vi "SPAN Stufen Gasteiler testen.vi"(5 "Stufen Tabelle Array":string[][][](array[string]), 6 "Sprachliste":string[][](array[string]), 7 "Boolsche Stufen Flags Cluster":T11, 8 "error in (no error)":errorcluster caption="Fehler (Eingang, kein Fehler)", 9 "Index":T13, 10 "Referenzen Cluster":T12, 11 "SpanInletClusterArray in":T2[](array[typedef]) {"zusätzliche Zeitdauer Erster Punkt" min=30 step=1 format="%#_5g"; "Zeitdauer Stufen" format="%#_5g"; "Max Fehler" format="%#_5g"; "Anzahl Stufen" format="%#_5g"; "Komponenten"."Komponente 5"."Komponente:" items=["NO (350,3000) LP 191C", "NO2 (150) LP 191C (1of2)", "NO2 (2000) LP 191C (2of2)", "N2O (300) LP 191C (1of2)", "NH3 (300) LP 191C (1of2)", "NH3 (900,3000) LP 191C (2of2)", "HNCO (400) 191C", "H2O% (30) LP 191C", "Formaldehyde (70,500) LP 191C", "CO2 low% (4) LP 191C (2of2)", "CO2% (20) LP 191C (1of2)", "CO (700) LP 191C (1of3)", "CO% (1) LP 191C (2of3)", "Propylene (1000) LP 191C", "Aromatic HC C7 (500) LP 191C", "Ethylene (1000) LP 191C", "CH4 (250) LP 191C (1of2)", "CH4 (5000) LP 191C (2of2)", "Ethane (1000) LP 191C", "Acetylene (1000) LP 191C", "HNO2 (20) 191C", "MeOH (1000) 191C", "CO% (10) LP 191C (3of3)", "Formic Acid (100) 191C", "SO2 (500) LP 191C", "Acetaldehyde (1000) LP 191C", "COS (100) LP 191C", "1,3 butadiene (100) LP 191C", "Oil as Octane (200) LP 191C", "N2O (1000) LP 191C (2of2)", "Propane (200) LP 191C", "NO2 autorange (2000)", "CO autorange (100000)", "CH4 autorange (5000)", "NH3 autorange (3000)", "Temp. Gascell", "Pressure Gascell", "sBeam@2500"]; "Komponenten"."Komponente 5"."Konzentration IST" format="%#.4f"; "Komponenten"."Komponente 5"."Genauigkeit" format="%#.1f"; "Komponenten"."Komponente 4"."Komponente:" items=["NO (350,3000) LP 191C", "NO2 (150) LP 191C (1of2)", "NO2 (2000) LP 191C (2of2)", "N2O (300) LP 191C (1of2)", "NH3 (300) LP 191C (1of2)", "NH3 (900,3000) LP 191C (2of2)", "HNCO (400) 191C", "H2O% (30) LP 191C", "Formaldehyde (70,500) LP 191C", "CO2 low% (4) LP 191C (2of2)", "CO2% (20) LP 191C (1of2)", "CO (700) LP 191C (1of3)", "CO% (1) LP 191C (2of3)", "Propylene (1000) LP 191C", "Aromatic HC C7 (500) LP 191C", "Ethylene (1000) LP 191C", "CH4 (250) LP 191C (1of2)", "CH4 (5000) LP 191C (2of2)", "Ethane (1000) LP 191C", "Acetylene (1000) LP 191C", "HNO2 (20) 191C", "MeOH (1000) 191C", "CO% (10) LP 191C (3of3)", "Formic Acid (100) 191C", "SO2 (500) LP 191C", "Acetaldehyde (1000) LP 191C", "COS (100) LP 191C", "1,3 butadiene (100) LP 191C", "Oil as Octane (200) LP 191C", "N2O (1000) LP 191C (2of2)", "Propane (200) LP 191C", "NO2 autorange (2000)", "CO autorange (100000)", "CH4 autorange (5000)", "NH3 autorange (3000)", "Temp. Gascell", "Pressure Gascell", "sBeam@2500"]; "Komponenten"."Komponente 4"."Konzentration IST" format="%#.4f"; "Komponenten"."Komponente 4"."Genauigkeit" format="%#.1f"; "Komponenten"."Komponente 3"."Komponente:" items=["NO (350,3000) LP 191C", "NO2 (150) LP 191C (1of2)", "NO2 (2000) LP 191C (2of2)", "N2O (300) LP 191C (1of2)", "NH3 (300) LP 191C (1of2)", "NH3 (900,3000) LP 191C (2of2)", "HNCO (400) 191C", "H2O% (30) LP 191C", "Formaldehyde (70,500) LP 191C", "CO2 low% (4) LP 191C (2of2)", "CO2% (20) LP 191C (1of2)", "CO (700) LP 191C (1of3)", "CO% (1) LP 191C (2of3)", "Propylene (1000) LP 191C", "Aromatic HC C7 (500) LP 191C", "Ethylene (1000) LP 191C", "CH4 (250) LP 191C (1of2)", "CH4 (5000) LP 191C (2of2)", "Ethane (1000) LP 191C", "Acetylene (1000) LP 191C", "HNO2 (20) 191C", "MeOH (1000) 191C", "CO% (10) LP 191C (3of3)", "Formic Acid (100) 191C", "SO2 (500) LP 191C", "Acetaldehyde (1000) LP 191C", "COS (100) LP 191C", "1,3 butadiene (100) LP 191C", "Oil as Octane (200) LP 191C", "N2O (1000) LP 191C (2of2)", "Propane (200) LP 191C", "NO2 autorange (2000)", "CO autorange (100000)", "CH4 autorange (5000)", "NH3 autorange (3000)", "Temp. Gascell", "Pressure Gascell", "sBeam@2500"]; "Komponenten"."Komponente 3"."Konzentration IST" format="%#.4f"; "Komponenten"."Komponente 3"."Genauigkeit" format="%#.1f"; "Komponenten"."Komponente 2"."Komponente:" items=["NO (350,3000) LP 191C", "NO2 (150) LP 191C (1of2)", "NO2 (2000) LP 191C (2of2)", "N2O (300) LP 191C (1of2)", "NH3 (300) LP 191C (1of2)", "NH3 (900,3000) LP 191C (2of2)", "HNCO (400) 191C", "H2O% (30) LP 191C", "Formaldehyde (70,500) LP 191C", "CO2 low% (4) LP 191C (2of2)", "CO2% (20) LP 191C (1of2)", "CO (700) LP 191C (1of3)", "CO% (1) LP 191C (2of3)", "Propylene (1000) LP 191C", "Aromatic HC C7 (500) LP 191C", "Ethylene (1000) LP 191C", "CH4 (250) LP 191C (1of2)", "CH4 (5000) LP 191C (2of2)", "Ethane (1000) LP 191C", "Acetylene (1000) LP 191C", "HNO2 (20) 191C", "MeOH (1000) 191C", "CO% (10) LP 191C (3of3)", "Formic Acid (100) 191C", "SO2 (500) LP 191C", "Acetaldehyde (1000) LP 191C", "COS (100) LP 191C", "1,3 butadiene (100) LP 191C", "Oil as Octane (200) LP 191C", "N2O (1000) LP 191C (2of2)", "Propane (200) LP 191C", "NO2 autorange (2000)", "CO autorange (100000)", "CH4 autorange (5000)", "NH3 autorange (3000)", "Temp. Gascell", "Pressure Gascell", "sBeam@2500"]; "Komponenten"."Komponente 2"."Konzentration IST" format="%#.4f"; "Komponenten"."Komponente 2"."Genauigkeit" format="%#.1f"; "Komponenten"."Komponente 1"."Komponente:" items=["NO (350,3000) LP 191C", "NO2 (150) LP 191C (1of2)", "NO2 (2000) LP 191C (2of2)", "N2O (300) LP 191C (1of2)", "NH3 (300) LP 191C (1of2)", "NH3 (900,3000) LP 191C (2of2)", "HNCO (400) 191C", "H2O% (30) LP 191C", "Formaldehyde (70,500) LP 191C", "CO2 low% (4) LP 191C (2of2)", "CO2% (20) LP 191C (1of2)", "CO (700) LP 191C (1of3)", "CO% (1) LP 191C (2of3)", "Propylene (1000) LP 191C", "Aromatic HC C7 (500) LP 191C", "Ethylene (1000) LP 191C", "CH4 (250) LP 191C (1of2)", "CH4 (5000) LP 191C (2of2)", "Ethane (1000) LP 191C", "Acetylene (1000) LP 191C", "HNO2 (20) 191C", "MeOH (1000) 191C", "CO% (10) LP 191C (3of3)", "Formic Acid (100) 191C", "SO2 (500) LP 191C", "Acetaldehyde (1000) LP 191C", "COS (100) LP 191C", "1,3 butadiene (100) LP 191C", "Oil as Octane (200) LP 191C", "N2O (1000) LP 191C (2of2)", "Propane (200) LP 191C", "NO2 autorange (2000)", "CO autorange (100000)", "CH4 autorange (5000)", "NH3 autorange (3000)", "Temp. Gascell", "Pressure Gascell", "sBeam@2500"]; "Komponenten"."Komponente 1"."Konzentration IST" format="%#.4f"; "Komponenten"."Komponente 1"."Genauigkeit" format="%#.1f"; "Ablaufdatum" format="%<%d.%m.%Y>T"; "Gasflasche" items=["----"=10000, "IAG NH3 3000"=0, "IAG NH3 200"=1, "IAG NH3 2000"=2, "IAG MG"=3, "IAG O2"=4]}) -> (0 "error out":errorcluster caption="Fehler (Ausgang)", 1 "GD LNI old or other":T1 caption="GD LNI old", 2 "GD DF":T1, 3 "SpanInletClusterArray out":T2[](array[typedef]) {"zusätzliche Zeitdauer Erster Punkt" min=30 step=1 format="%#_5g"; "Zeitdauer Stufen" format="%#_5g"; "Max Fehler" format="%#_5g"; "Anzahl Stufen" format="%#_5g"; "Komponenten"."Komponente 5"."Komponente:" items=["NO (350,3000) LP 191C", "NO2 (150) LP 191C (1of2)", "NO2 (2000) LP 191C (2of2)", "N2O (300) LP 191C (1of2)", "NH3 (300) LP 191C (1of2)", "NH3 (900,3000) LP 191C (2of2)", "HNCO (400) 191C", "H2O% (30) LP 191C", "Formaldehyde (70,500) LP 191C", "CO2 low% (4) LP 191C (2of2)", "CO2% (20) LP 191C (1of2)", "CO (700) LP 191C (1of3)", "CO% (1) LP 191C (2of3)", "Propylene (1000) LP 191C", "Aromatic HC C7 (500) LP 191C", "Ethylene (1000) LP 191C", "CH4 (250) LP 191C (1of2)", "CH4 (5000) LP 191C (2of2)", "Ethane (1000) LP 191C", "Acetylene (1000) LP 191C", "HNO2 (20) 191C", "MeOH (1000) 191C", "CO% (10) LP 191C (3of3)", "Formic Acid (100) 191C", "SO2 (500) LP 191C", "Acetaldehyde (1000) LP 191C", "COS (100) LP 191C", "1,3 butadiene (100) LP 191C", "Oil as Octane (200) LP 191C", "N2O (1000) LP 191C (2of2)", "Propane (200) LP 191C", "NO2 autorange (2000)", "CO autorange (100000)", "CH4 autorange (5000)", "NH3 autorange (3000)", "Temp. Gascell", "Pressure Gascell", "sBeam@2500"]; "Komponenten"."Komponente 5"."Konzentration IST" format="%#.4f"; "Komponenten"."Komponente 5"."Genauigkeit" format="%#.1f"; "Komponenten"."Komponente 4"."Komponente:" items=["NO (350,3000) LP 191C", "NO2 (150) LP 191C (1of2)", "NO2 (2000) LP 191C (2of2)", "N2O (300) LP 191C (1of2)", "NH3 (300) LP 191C (1of2)", "NH3 (900,3000) LP 191C (2of2)", "HNCO (400) 191C", "H2O% (30) LP 191C", "Formaldehyde (70,500) LP 191C", "CO2 low% (4) LP 191C (2of2)", "CO2% (20) LP 191C (1of2)", "CO (700) LP 191C (1of3)", "CO% (1) LP 191C (2of3)", "Propylene (1000) LP 191C", "Aromatic HC C7 (500) LP 191C", "Ethylene (1000) LP 191C", "CH4 (250) LP 191C (1of2)", "CH4 (5000) LP 191C (2of2)", "Ethane (1000) LP 191C", "Acetylene (1000) LP 191C", "HNO2 (20) 191C", "MeOH (1000) 191C", "CO% (10) LP 191C (3of3)", "Formic Acid (100) 191C", "SO2 (500) LP 191C", "Acetaldehyde (1000) LP 191C", "COS (100) LP 191C", "1,3 butadiene (100) LP 191C", "Oil as Octane (200) LP 191C", "N2O (1000) LP 191C (2of2)", "Propane (200) LP 191C", "NO2 autorange (2000)", "CO autorange (100000)", "CH4 autorange (5000)", "NH3 autorange (3000)", "Temp. Gascell", "Pressure Gascell", "sBeam@2500"]; "Komponenten"."Komponente 4"."Konzentration IST" format="%#.4f"; "Komponenten"."Komponente 4"."Genauigkeit" format="%#.1f"; "Komponenten"."Komponente 3"."Komponente:" items=["NO (350,3000) LP 191C", "NO2 (150) LP 191C (1of2)", "NO2 (2000) LP 191C (2of2)", "N2O (300) LP 191C (1of2)", "NH3 (300) LP 191C (1of2)", "NH3 (900,3000) LP 191C (2of2)", "HNCO (400) 191C", "H2O% (30) LP 191C", "Formaldehyde (70,500) LP 191C", "CO2 low% (4) LP 191C (2of2)", "CO2% (20) LP 191C (1of2)", "CO (700) LP 191C (1of3)", "CO% (1) LP 191C (2of3)", "Propylene (1000) LP 191C", "Aromatic HC C7 (500) LP 191C", "Ethylene (1000) LP 191C", "CH4 (250) LP 191C (1of2)", "CH4 (5000) LP 191C (2of2)", "Ethane (1000) LP 191C", "Acetylene (1000) LP 191C", "HNO2 (20) 191C", "MeOH (1000) 191C", "CO% (10) LP 191C (3of3)", "Formic Acid (100) 191C", "SO2 (500) LP 191C", "Acetaldehyde (1000) LP 191C", "COS (100) LP 191C", "1,3 butadiene (100) LP 191C", "Oil as Octane (200) LP 191C", "N2O (1000) LP 191C (2of2)", "Propane (200) LP 191C", "NO2 autorange (2000)", "CO autorange (100000)", "CH4 autorange (5000)", "NH3 autorange (3000)", "Temp. Gascell", "Pressure Gascell", "sBeam@2500"]; "Komponenten"."Komponente 3"."Konzentration IST" format="%#.4f"; "Komponenten"."Komponente 3"."Genauigkeit" format="%#.1f"; "Komponenten"."Komponente 2"."Komponente:" items=["NO (350,3000) LP 191C", "NO2 (150) LP 191C (1of2)", "NO2 (2000) LP 191C (2of2)", "N2O (300) LP 191C (1of2)", "NH3 (300) LP 191C (1of2)", "NH3 (900,3000) LP 191C (2of2)", "HNCO (400) 191C", "H2O% (30) LP 191C", "Formaldehyde (70,500) LP 191C", "CO2 low% (4) LP 191C (2of2)", "CO2% (20) LP 191C (1of2)", "CO (700) LP 191C (1of3)", "CO% (1) LP 191C (2of3)", "Propylene (1000) LP 191C", "Aromatic HC C7 (500) LP 191C", "Ethylene (1000) LP 191C", "CH4 (250) LP 191C (1of2)", "CH4 (5000) LP 191C (2of2)", "Ethane (1000) LP 191C", "Acetylene (1000) LP 191C", "HNO2 (20) 191C", "MeOH (1000) 191C", "CO% (10) LP 191C (3of3)", "Formic Acid (100) 191C", "SO2 (500) LP 191C", "Acetaldehyde (1000) LP 191C", "COS (100) LP 191C", "1,3 butadiene (100) LP 191C", "Oil as Octane (200) LP 191C", "N2O (1000) LP 191C (2of2)", "Propane (200) LP 191C", "NO2 autorange (2000)", "CO autorange (100000)", "CH4 autorange (5000)", "NH3 autorange (3000)", "Temp. Gascell", "Pressure Gascell", "sBeam@2500"]; "Komponenten"."Komponente 2"."Konzentration IST" format="%#.4f"; "Komponenten"."Komponente 2"."Genauigkeit" format="%#.1f"; "Komponenten"."Komponente 1"."Komponente:" items=["NO (350,3000) LP 191C", "NO2 (150) LP 191C (1of2)", "NO2 (2000) LP 191C (2of2)", "N2O (300) LP 191C (1of2)", "NH3 (300) LP 191C (1of2)", "NH3 (900,3000) LP 191C (2of2)", "HNCO (400) 191C", "H2O% (30) LP 191C", "Formaldehyde (70,500) LP 191C", "CO2 low% (4) LP 191C (2of2)", "CO2% (20) LP 191C (1of2)", "CO (700) LP 191C (1of3)", "CO% (1) LP 191C (2of3)", "Propylene (1000) LP 191C", "Aromatic HC C7 (500) LP 191C", "Ethylene (1000) LP 191C", "CH4 (250) LP 191C (1of2)", "CH4 (5000) LP 191C (2of2)", "Ethane (1000) LP 191C", "Acetylene (1000) LP 191C", "HNO2 (20) 191C", "MeOH (1000) 191C", "CO% (10) LP 191C (3of3)", "Formic Acid (100) 191C", "SO2 (500) LP 191C", "Acetaldehyde (1000) LP 191C", "COS (100) LP 191C", "1,3 butadiene (100) LP 191C", "Oil as Octane (200) LP 191C", "N2O (1000) LP 191C (2of2)", "Propane (200) LP 191C", "NO2 autorange (2000)", "CO autorange (100000)", "CH4 autorange (5000)", "NH3 autorange (3000)", "Temp. Gascell", "Pressure Gascell", "sBeam@2500"]; "Komponenten"."Komponente 1"."Konzentration IST" format="%#.4f"; "Komponenten"."Komponente 1"."Genauigkeit" format="%#.1f"; "Ablaufdatum" format="%<%d.%m.%Y>T"; "Gasflasche" items=["----"=10000, "IAG NH3 3000"=0, "IAG NH3 200"=1, "IAG NH3 2000"=2, "IAG MG"=3, "IAG O2"=4]})   [LabVIEW 2020, in "Linearisierung v2.lvlib" / "SpanEinstellungen.lvlib"]
uses:
  SpanEinstellungen.lvlib
  GD Abfrage Referenzen.ctl
  Boolsche Stufen Flags.ctl
  SpanInletCluster.ctl
  Seiten/System Einstellungen V2/Konfig Gasflasche.ctl
  Seiten/System Einstellungen V2/Analysatoren.ctl
  Seiten/System Einstellungen V2/Gasflasche Auswahl.ctl
  Komponentencluster mit Formel.ctl
  Komponentenauswahl mit Formel.ctl
  Visualisierungs Elemente/String - Eingabefeld.ctl
  Einheit.ctl
  Seiten/System Einstellungen V2/Traegergas.ctl
  Visualisierungs Elemente/Checkbox(boolsch).ctl
  Gasteiler/Aktionen FGV Gasteiler Daten.ctl
  GasteilerType.ctl
  Linearisierung v2.lvlib
  Gasteiler/Gasteiler.lvlib
  Sprachverwaltung/Sprachverwaltung.lvlib
  Seiten/System Einstellungen V2/System Einstellungen V2.lvlib
panel:
  # "sec"
  # "%"
  # "sec"
  # "Komponente"
  # "Formel"
  # "Konzentration"
  # "Einheit"
  # "Genauigkeit [%]"
  # "sec"
  # "%"
  # "sec"
  # "Komponente"
  # "Formel"
  # "Konzentration"
  # "Einheit"
  # "Genauigkeit [%]"
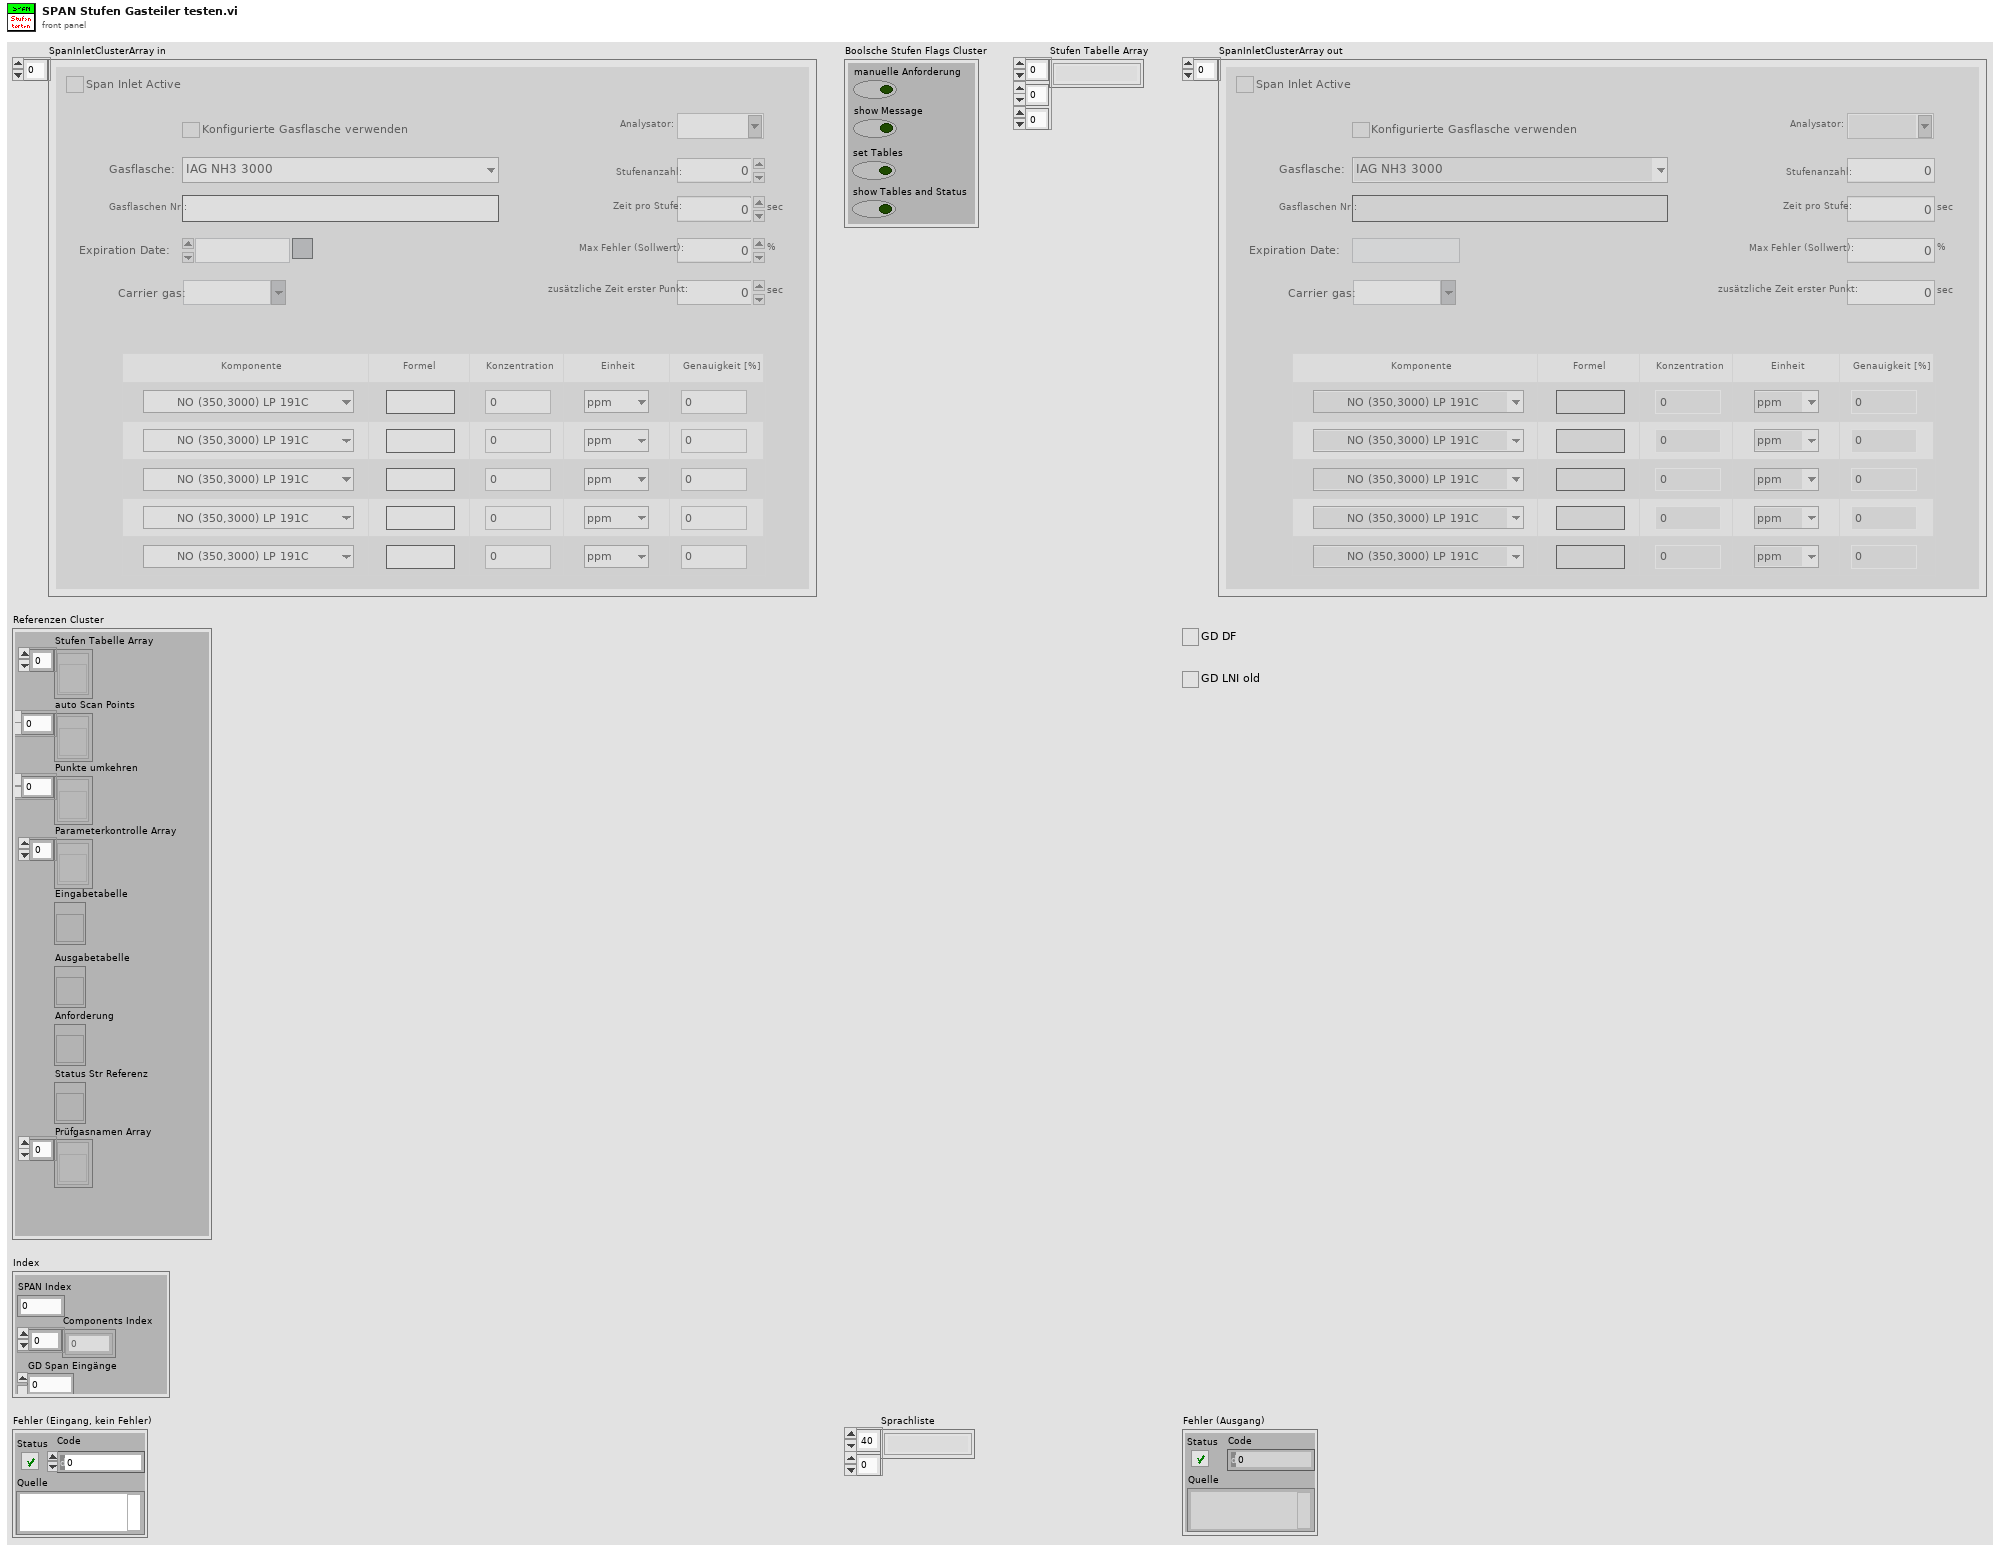
[diagram p1: front panel]
types:
  T1 = typedef "Checkbox(boolsch).ctl" = bool
  T2 = typedef "Linearisierung v2.lvlib/SpanEinstellungen.lvlib/SpanInletCluster.ctl" = cluster{"Span Inlet Active":T3, "Analysator":T4, "Konfig Gasflasche":T3, "Gasflasche":T5, "Gasflaschen Nr.:":string, "Ablaufdatum":timestamp, "Komponenten":T6, "Zeitdauer Stufen":sgl, "Max Fehler":sgl, "Anzahl Stufen":sgl, "Trägergas":T10, "zusätzliche Zeitdauer Erster Punkt":sgl}
  T3 = typedef "System Einstellungen V2.lvlib/Konfig Gasflasche.ctl" = bool
  T4 = typedef "System Einstellungen V2.lvlib/Analysatoren.ctl" = string
  T5 = typedef "System Einstellungen V2.lvlib/Gasflasche Auswahl.ctl" = u16
  T6 = typedef "Linearisierung v2.lvlib/SpanEinstellungen.lvlib/Komponentencluster mit Formel.ctl" = cluster{"Komponente 1":T7, "Komponente 2":T7, "Komponente 3":T7, "Komponente 4":T7, "Komponente 5":T7}
  T7 = typedef "Linearisierung v2.lvlib/SpanEinstellungen.lvlib/Komponentenauswahl mit Formel.ctl" = cluster{"Komponente:":u16, "Summenformel":T8, "Konzentration IST":dbl, "Einheit":T9, "Genauigkeit":dbl}
  T8 = typedef "String - Eingabefeld.ctl" = string
  T9 = typedef "Linearisierung v2.lvlib/SpanEinstellungen.lvlib/Einheit.ctl" = enum16{"ppm", "%"}
  T10 = typedef "System Einstellungen V2.lvlib/Traegergas.ctl" = string
  T11 = typedef "Linearisierung v2.lvlib/SpanEinstellungen.lvlib/Boolsche Stufen Flags.ctl" = cluster{"manuelle Anforderung":bool, "show Message":bool, "set Tables":bool, "show Tables and Status":bool}
  T12 = typedef "Linearisierung v2.lvlib/SpanEinstellungen.lvlib/GD Abfrage Referenzen.ctl" = cluster{"Stufen Tabelle Array":refnum<vi>[], "auto Scan Points":refnum<vi>[], "Punkte umkehren":refnum<vi>[], "Parameterkontrolle Array":refnum<vi>[], "Eingabetabelle":refnum<vi>, "Ausgabetabelle":refnum<vi>, "Anforderung":refnum<vi>, "Status Str Referenz":refnum<vi>, "Prüfgasnamen Array":refnum<vi>[]}
  T13 = cluster{"SPAN Index":i32, "Components Index":i32[], "GD Span Eingänge":u16}
  T14 = typedef "Linearisierung v2.lvlib/GasteilerType.ctl" = u16
  T15 = typedef "Linearisierung v2.lvlib/Gasteiler.lvlib/Aktionen FGV Gasteiler Daten.ctl" = enum16{"lesen", "Gasteiler Daten", "Seriellen Param.", "MB-Endwert", "laden", "speichern", "Anforderung", "TCP", "Aufzeichnung Start"}
  T16 = typedef "Linearisierung v2.lvlib/Gasteiler.lvlib/Gasteiler Daten.ctl" = cluster{"Gasteiler":T8, "Gasteiler Stufen":T17, "Gasteiler Type":T14, "Konfig Gasteiler":T18, "Gasteiler Span Eingänge":u16}
  T17 = typedef "Linearisierung v2.lvlib/Gasteiler.lvlib/Gasteiler Stufen.ctl" = u16
  T18 = typedef "System Einstellungen V2.lvlib/Gasteiler Auswahl.ctl" = u16
  T19 = typedef "Button.ctl" = bool
  T20 = cluster{"Komponente:":u16, "Konzentration IST":dbl}[]
  T21 = typedef "Linearisierung v2.lvlib/Gasteiler.lvlib/Prüfgas in.ctl" = u16
  T22 = cluster{"Anzahl Stufen":sgl, "Verdünnungsgas":T21, "Components Index":i32[]}
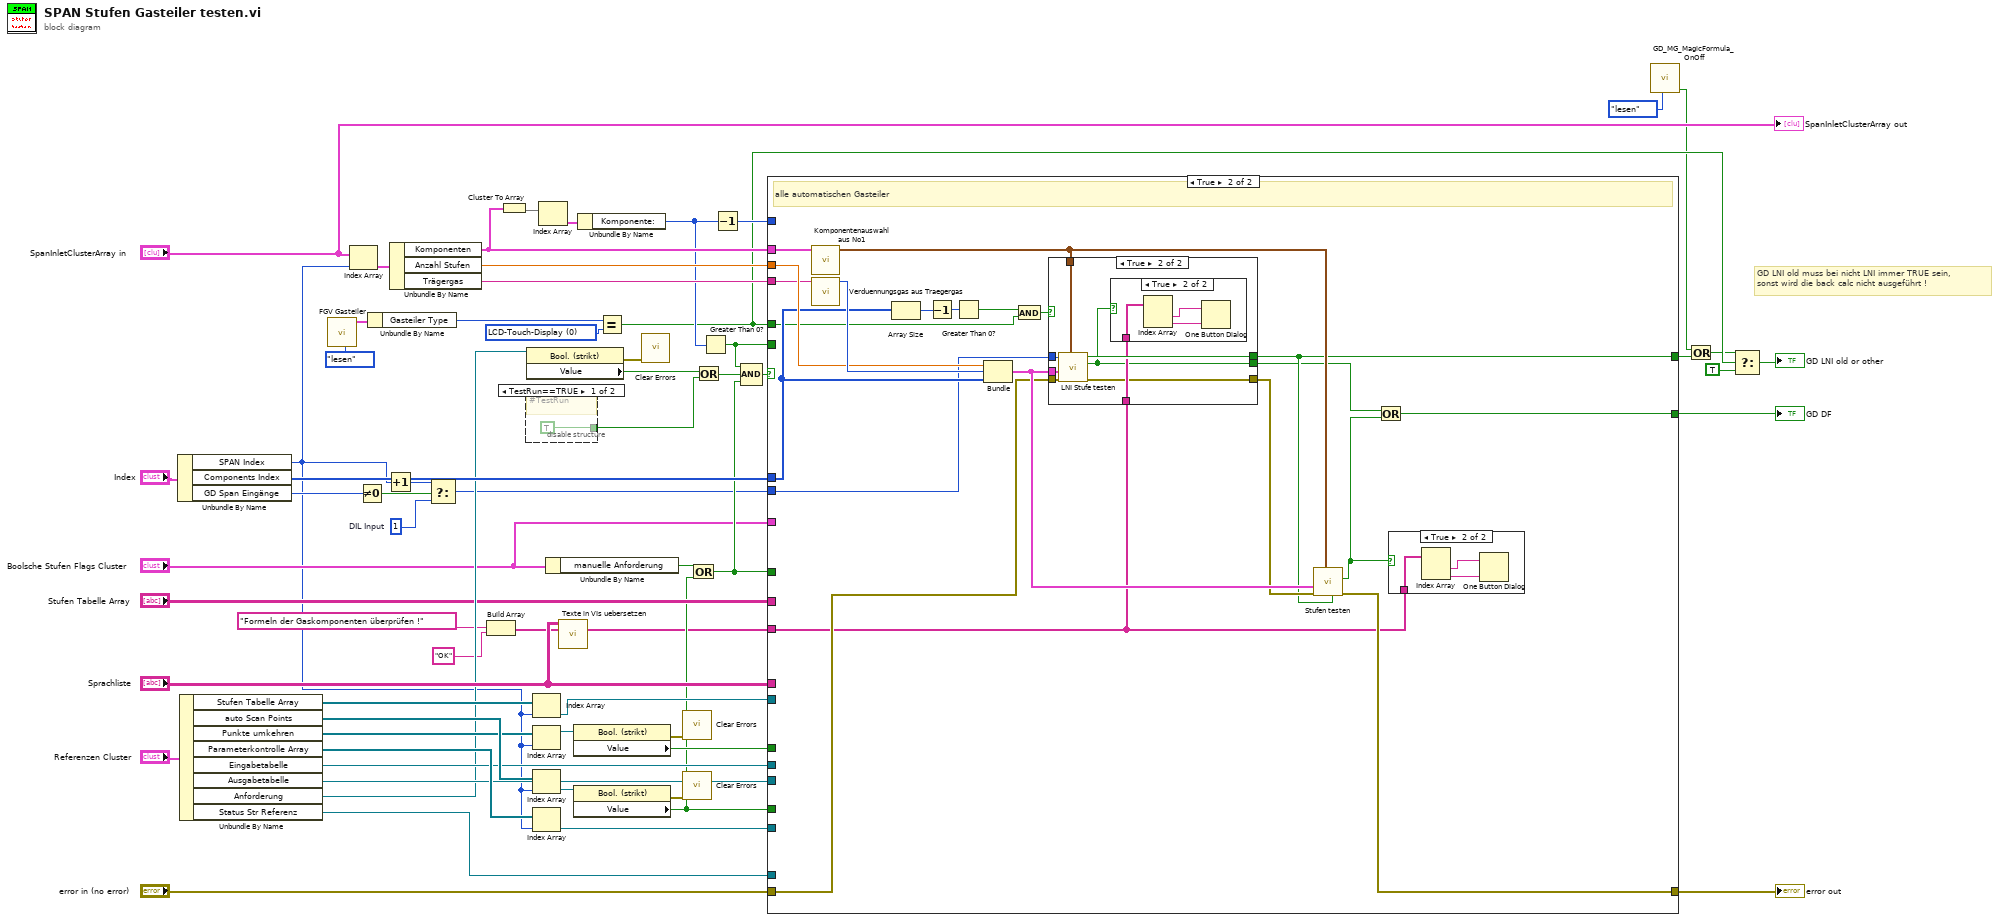
[diagram p0: block diagram]
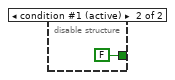
[diagram p2: hidden frame]
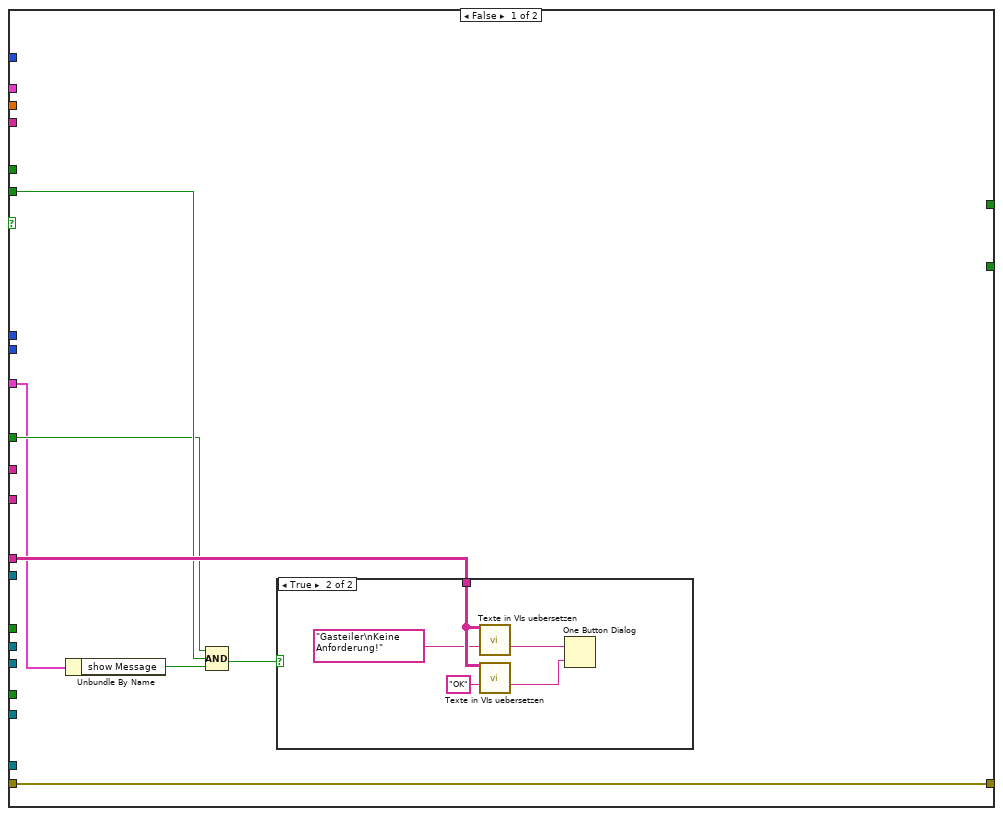
[diagram p3: hidden frame]
diagram:
  w8 = 1  # DIL Input
  w15 = T14 0 items=["LCD-Touch-Display", "Analog-Display", "AVL GDU", "Horiba GDC", "HovaCal", "Horiba 710 c"] ("x")
  # "GD LNI old muss bei nicht LNI immer TRUE sein,\nsonst wird die back calc nicht ausgeführt !"
  n1 = Unbundle By Name("Index") -> ("SPAN Index"=w4:i32, "Components Index"=w56:i32[], "GD Span Eingänge"=w5:u16)
  n2 = Unbundle By Name("Referenzen Cluster") -> ("Stufen Tabelle Array"=w54:refnum<vi>[], "auto Scan Points"=w53:refnum<vi>[], "Punkte umkehren"=w52:refnum<vi>[], "Parameterkontrolle Array"=w51:refnum<vi>[], "Eingabetabelle"=w50:refnum<vi>, "Ausgabetabelle"=w39:refnum<vi>, "Anforderung"=w37:refnum<vi>, "Status Str Referenz"=w38:refnum<vi>)
  n3 = call "FGV Gasteiler.vi"("Aktionen"=Aktionen_FGV_Gasteiler_Daten."lesen") -> ("Gasteiler Daten"=w61:T16)  [unwired: 11 in, 7 out]
  n4 = Index Array(array="SpanInletClusterArray in", index=w4) -> (element=w33:T2)
  n5 = Not Equal To 0?(x=w5) -> (x != 0?=w9:bool)
  n6 = Unbundle By Name(w61) -> ("Gasteiler Type"=w14:T14)
  n7 = Increment(x=w4) -> (x+1=w7:i32)
  n8 = Unbundle By Name(w33) -> ("Komponenten"=w30:T6, "Anzahl Stufen"=w32:sgl, "Trägergas"=w31:T10)
  n9 = Select(t=w7, s=w9, f=w8) -> (s? t:f=w6:i32)
  n10 = Build Array("Formeln der Gaskomponenten überprüfen !" ("Nachricht"), "OK" ("String zum Übersetzen")) -> (w19:string[])
  n11 = Cluster To Array(cluster=w30) -> (array=w34:T7[])
  n12 = disable-structure shown="TestRun==TRUE" {
    disable-tunnel: [TRUE FALSE] -> w40
    frame condition #0 {
      # "#TestRun"
    }
    frame condition #1 (active) {
    }
  }
  n13 = property class="Bool. (strikt)"(reference=w37) -> (error out=w45:errorcluster, "Value"=w46:T19)  [unwired: 1 in, 1 out]
  n14 = Index Array(array=w54, index=w4) -> (element=w44:refnum<vi>)
  n15 = Index Array(array=w52, index=w4) -> (element=w60:refnum<vi>)
  n16 = Index Array(array=w53, index=w4) -> (element=w48:refnum<vi>)
  n17 = Index Array(array=w51, index=w4) -> (element=w63:refnum<vi>)
  n18 = Index Array(array=w34) -> (element=w35:T7)  [unwired: 1 in]
  n19 = Unbundle By Name("Boolsche Stufen Flags Cluster") -> ("manuelle Anforderung"=w24:bool)
  n20 = call "Texte in VIs uebersetzen.vi"("Sprachliste"="Sprachliste", "String-Array zum Übersetzen"=w19) -> ("String-Array zum Übersetzen"=w18:string[])  [unwired: 9 in, 4 out]
  n21 = property class="Bool. (strikt)"(reference=w60) -> (error out=w58:errorcluster, "Value"=w59:bool)  [unwired: 1 in, 1 out]
  n22 = property class="Bool. (strikt)"(reference=w48) -> (error out=w49:errorcluster, "Value"=w23:bool)  [unwired: 1 in, 1 out]
  n23 = Unbundle By Name(w35) -> ("Komponente:"=w27:u16)
  n24 = Equal?(x=w14, y=w15) -> (x = y?=w13:bool)
  n25 = call <vilib>:"Clear Errors.vi"("error in (no error)"=w45) -> ()  [unwired: 5 in, 2 out]
  n26 = call <vilib>:"Clear Errors.vi"("error in (no error)"=w58) -> ()  [unwired: 5 in, 2 out]
  n27 = call <vilib>:"Clear Errors.vi"("error in (no error)"=w49) -> ()  [unwired: 5 in, 2 out]
  n28 = Or(x=w24, y=w23) -> (x .or. y?=w22:bool)
  n29 = Or(x=w46, y=w40) -> (x .or. y?=w41:T19)
  n30 = Greater Than 0?(x=w27) -> (x > 0?=w26:bool)
  n31 = Decrement(x=w27) -> (x-1=w28:u16)
  n32 = Compound Arithmetic op=AND ("Mehrfacharithmetik")(w26, w41, w22) -> (w29:T19)
  n33 = case shown="True" w29 {
    tunnel: w63 -> [_ _]
    tunnel: w50 -> [_ _]
    tunnel: w59 -> [_ _]
    tunnel: w56 -> [_ w93]
    tunnel: w23 -> [_ _]
    tunnel: "Sprachliste" -> [w72 _]
    tunnel: w44 -> [_ _]
    tunnel: "error in (no error)" -> [w71 w87]
    tunnel: [w71 w94] -> w42
    tunnel: w38 -> [_ _]
    tunnel: w39 -> [_ _]
    tunnel: w30 -> [_ w97]
    tunnel: w32 -> [_ w96]
    tunnel: w31 -> [_ w95]
    tunnel: w28 -> [_ _]
    tunnel: w26 -> [w68 _]
    tunnel: "Stufen Tabelle Array" -> [_ _]
    tunnel: w22 -> [w67 _]
    tunnel: w18 -> [_ w84]
    tunnel: [_ w83] -> w10
    tunnel: "Boolsche Stufen Flags Cluster" -> [w66 _]
    tunnel: [_ w80] -> w16
    tunnel: w13 -> [_ w79]
    tunnel: w6 -> [_ w78]
    frame False {
      n34 = Unbundle By Name(w66) -> ("show Message"=w70:bool)
      n35 = Compound Arithmetic op=AND ("Mehrfacharithmetik")(w67, w68, w70) -> (w69:bool)
      n36 = case shown="True" w69 {
        tunnel: w72 -> [_ w77]
        frame False {
        }
        frame True {
          n37 = call "Texte in VIs uebersetzen.vi"("Sprachliste"=w77, "String zum Übersetzen"="Gasteiler\nKeine Anforderung!" ("Nachricht")) -> ("String zum Übersetzen"=w75:string)  [unwired: 9 in, 4 out]
          n38 = call "Texte in VIs uebersetzen.vi"("Sprachliste"=w77, "String zum Übersetzen"="OK") -> ("String zum Übersetzen"=w74:string)  [unwired: 9 in, 4 out]
          n39 = One Button Dialog(message=w75, button name ("OK")=w74) -> ()  [unwired: 1 out]
        }
      }
    }
    frame True {
      # "alle automatischen Gasteiler"
      n40 = call "Komponentenauswahl aus No1.vi"("Komponente 1"=w97) -> ("Komponentenauswahl"=w89:T20)  [unwired: 8 in, 2 out]
      n41 = call "Verduennungsgas aus Traegergas.vi"("Trägergas"=w95) -> ("Verdünnungsgas"=w98:T21)  [unwired: 10 in]
      n42 = Array Size(array=w93) -> (size(s)=w92:i32)
      n43 = Decrement(x=w92) -> (x-1=w85:i32)
      n44 = Greater Than 0?(x=w85) -> (x > 0?=w91:bool)
      n45 = Bundle("Anzahl Stufen"=w96, "Verdünnungsgas"=w98, "Components Index"=w93) -> (w88:T22)  [unwired: 1 in]
      n46 = And(x=w91, y=w79) -> (x .and. y?=w90:bool)
      n47 = case shown="True" w90 {
        tunnel: w89 -> [_ w110]
        tunnel: w88 -> [_ w109]
        tunnel: [_ w108] -> w83
        tunnel: w84 -> [_ w107]
        tunnel: w87 -> [w102 w106]
        tunnel: [w102 w105] -> w86
        tunnel: [_ w104] -> w82
        tunnel: w78 -> [_ w103]
        frame False {
        }
        frame True {
          n48 = call "LNI Stufe testen.vi"("Komponentenauswahl"=w110, "error in (no error)"=w106, "Index Cluster"=w109, "GD DIL Input"=w103) -> ("error out"=w105:errorcluster, "GD DF"=w104:T1, "GD LNI old"=w108:T1)  [unwired: 5 in]
          n49 = case shown="True" w104 {
            tunnel: w107 -> [_ w113]
            frame False {
            }
            frame True {
              n50 = Index Array(array=w113) -> (element #1=w112:string, element #2=w111:string)  [unwired: 2 in]
              n51 = One Button Dialog(message=w112, button name ("OK")=w111) -> ()  [unwired: 1 out]
            }
          }
        }
      }
      n52 = call "Stufen testen.vi"("GD LNI old"=w83, "Komponentenauswahl"=w89, "error in (no error)"=w86, "Index Cluster"=w88) -> ("error out"=w94:errorcluster, "GD DF"=w81:T1)  [unwired: 6 in]
      n53 = Or(x=w82, y=w81) -> (x .or. y?=w80:T1)
      n54 = case shown="True" w81 {
        tunnel: w84 -> [_ w101]
        frame False {
        }
        frame True {
          n55 = Index Array(array=w101) -> (element #1=w100:string, element #2=w99:string)  [unwired: 2 in]
          n56 = One Button Dialog(message=w100, button name ("OK")=w99) -> ()  [unwired: 1 out]
        }
      }
    }
  }
  "error out" <- w42
  "GD DF" <- w16
  n57 = call "GD_MG_MagicFormula_OnOff.vi"("Aktion"=enum16{"lesen", "schreiben", "init"}."lesen") -> ("use old LNI"=w1:bool)  [unwired: 8 in, 1 out]
  n58 = Or(x=w1, y=w10) -> (x .or. y?=w2:T1)
  n59 = Select(t=w2, s=w13, f=T3 TRUE) -> (s? t:f=→"GD LNI old or other":T3)
  "SpanInletClusterArray out" <- "SpanInletClusterArray in"
